vi "Blink.vi"(8 "error in (no error)":errorcluster, 11 "milliseconds to wait (100)":u32=100) -> (0 "error out":errorcluster)   [LabVIEW 2015]
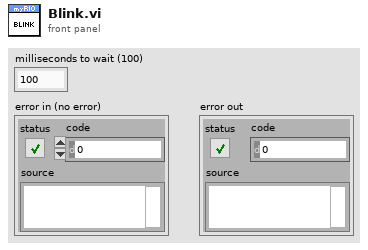
[diagram p1: front panel]
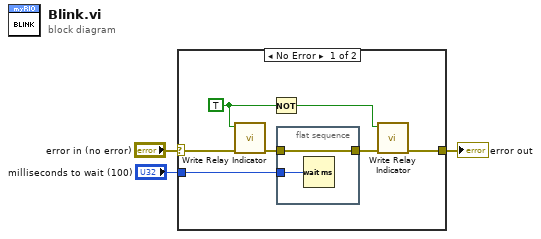
[diagram p0: block diagram]
diagram:
  n1 = case shown="No Error" "error in (no error)" {
    selector: "error in (no error)" -> [w7 w13]
    tunnel: [w4 w13] -> w3
    tunnel: "milliseconds to wait (100)" -> [w10 _]
    frame No Error {
      w8 = TRUE ("Relay")
      n2 = call "Write Relay Indicator.vi"("error in (no error)"=w7, "status"=w8) -> ("error out"=w5:errorcluster)  [unwired: 9 in]
      n3 = Not(x=w8) -> (.not. x?=w9:bool)
      n4 = flat-sequence {
        tunnel: w10 -> [w12]
        tunnel: [w11] -> w6
        tunnel: w5 -> [w11]
        frame #0 {
          n5 = Wait (ms)(milliseconds to wait=w12) -> ()  [unwired: 1 out]
        }
      }
      n6 = call "Write Relay Indicator.vi"("error in (no error)"=w6, "status"=w9) -> ("error out"=w4:errorcluster)  [unwired: 9 in]
    }
    frame Error {
    }
  }
  "error out" <- w3
